vi "Write_Axis_Pos_tl.vi"(2 "Position":dbl format="%.5f", 3 "Axis":string) -> (0 "Index":i32, 1 "Axis Position Cluster":T1 {"mac position" format="%.5f"})   [LabVIEW 2010]
doc: "Writes to the channel positions array of the traverse setup global"
uses:
  Custom Controls/Axis_pos_cluster_tl.ctl
  Traverse_setup_tl.glob.vi
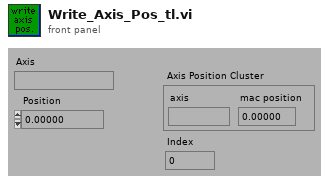
[diagram p1: front panel]
types:
  T1 = typedef "Axis_pos_cluster_tl.ctl" = cluster{"axis":string, "mac position":dbl}
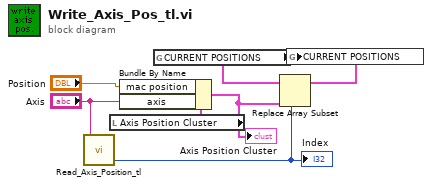
[diagram p0: block diagram]
diagram:
  n1 = call "Read_Axis_Position_tl.vi"("Axis"="Axis") -> ("Index"=w2:i32)  [unwired: 1 out]
  "Index" <- w2
  n2 = local read "Axis Position Cluster"() -> (w5:T1)
  n3 = Bundle By Name(cluster=w5, "mac position"="Position", "axis"="Axis") -> (w4:T1)
  "Axis Position Cluster" <- w4
  n4 = global read "Traverse_setup_tl.glob.vi" "CURRENT POSITIONS"() -> (w6:T1[])
  n5 = Replace Array Subset(array=w6, new element=w4, index=w2) -> (w7:T1[])
  n6 = global write "Traverse_setup_tl.glob.vi" "CURRENT POSITIONS"(w7) -> ()
